vi "Localize_Particles-10.vi"(5 "Keep Nega-\ntive Values?":bool, 7 "error IN":errorcluster, 8 "[IN] Sigma":dbl min=0.1, 9 "[IN] Destination Image":T1, 10 "[IN] Frame":T1) -> (0 "error OUT":errorcluster, 2 "[OUT] Histogram Graph":T2 {"Incremental Value" format="%.2f"; "Starting Value" format="%.2f"}, 3 "[OUT] LoG Processed Image":T1)   [LabVIEW 2013]
doc: "Performing the LoG image processing\nWithout gamma correction initial (implemented explicitly before)"
uses:
  <vilib>/vision/Image Controls.llb/IMAQ Image.ctl
  <vilib>/vision/NI_Vision_Development_Module.lvlib
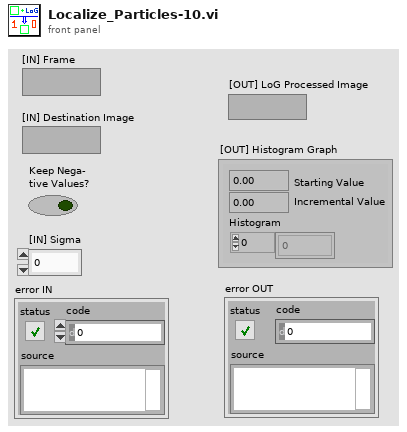
[diagram p1: front panel]
types:
  T1 = typedef "IMAQ Image.ctl" = refnum<image>
  T2 = cluster{"Starting Value":sgl, "Incremental Value":sgl, "Histogram":u32[]}
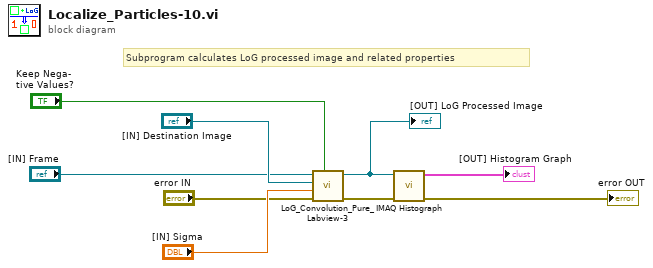
[diagram p0: block diagram]
diagram:
  # "Subprogram calculates LoG processed image and related properties"
  n1 = call "LoG_Convolution_Pure_Labview-3.vi"("Keep Nega-\ntive Values?"="Keep Nega-\ntive Values?", "error IN"="error IN", "[IN] Sigma"="[IN] Sigma", "[IN] Processed Image"="[IN] Destination Image", "[IN] Source Image"="[IN] Frame") -> ("error out"=w4:errorcluster, "[OUT] Processed Image"=w3:T1)  [unwired: 2 in]
  "[OUT] LoG Processed Image" <- w3
  n2 = call "IMAQ Histograph"("error in (no error)"=w4, "Image"=w3) -> ("error out"=→"error OUT":errorcluster, "Histogram Graph"=→"[OUT] Histogram Graph":T2)  [unwired: 6 in, 2 out]
